vi "Open Hardware.vi"(8 "error in (no error)":errorcluster, 11 "Inst.Krohn-Hite-7008 in":refnum<class "Inst.Krohn-Hite-7008.lvclass">) -> (0 "error out":errorcluster, 3 "Inst.Krohn-Hite-7008 out":refnum<class "Inst.Krohn-Hite-7008.lvclass">)   [LabVIEW 2019, in "Inst.Krohn-Hite-7008.lvclass"]
uses:
  Inst.Krohn-Hite-7008.lvclass
  C:/Program Files (x86)/National Instruments/LabVIEW 2019/user.lib/LevyLab/Instrument Framework/SMOs/Instrument/Instrument.lvclass
  Inst.Krohn-Hite-7008.lvclass/Inst.Krohn-Hite-7008.ctl
  <userlib>/LevyLab/Instrument Framework/SMOs/Instrument/Instrument.lvclass/Instrument.ctl
  <userlib>/LevyLab/Instrument Framework/Instrument Types/VSource/Instrument.VSource.lvclass
  <userlib>/LevyLab/Instrument Framework/SMOs/Instrument/Instrument.lvclass
  <userlib>/LevyLab/D2XX-LV/D2XX-lv.lvlib
  KH7008/KH7008.lvlib
  C:/Program Files (x86)/National Instruments/LabVIEW 2019/user.lib/LevyLab/Instrument Framework/Instrument Types/VSource/Instrument.VSource.lvclass
  C:/Program Files (x86)/National Instruments/LabVIEW 2019/vi.lib/JKI/JKI SMO/SMO/SMO.lvclass
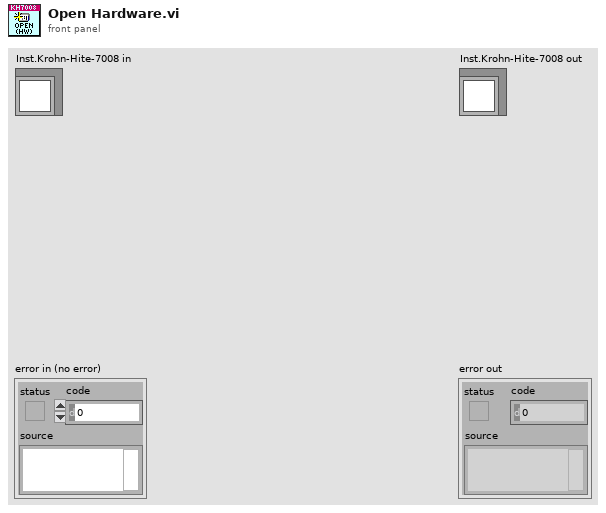
[diagram p1: front panel]
types:
  T1 = typedef "D2XX-lv.lvlib/Device Info.ctl" = cluster{"Serial Number":string, "COM port":string, "Description":string}
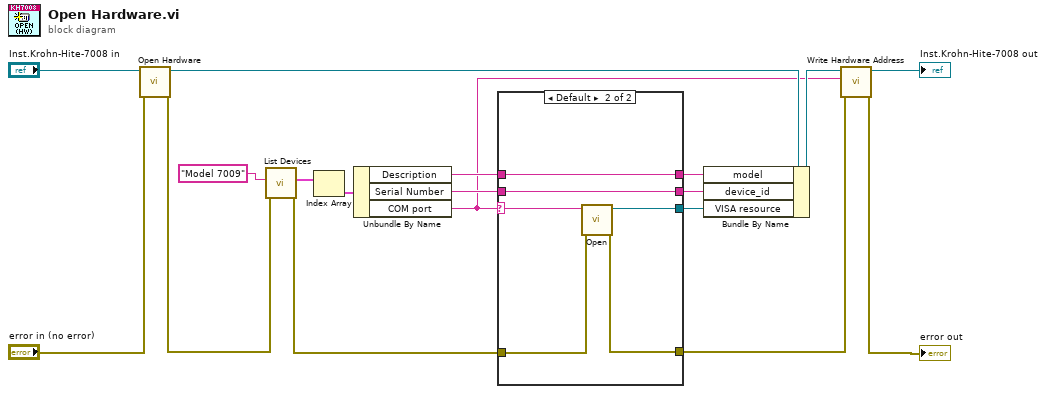
[diagram p0: block diagram]
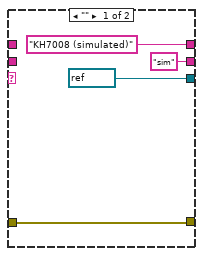
[diagram p2: hidden frame]
diagram:
  n1 = call-parent "Open Hardware.vi"("error in (no error)"="error in (no error)", "Instrument in"="Inst.Krohn-Hite-7008 in") -> ("error out"=w13:errorcluster, "Instrument out"=w16:refnum<class "Inst.Krohn-Hite-7008.lvclass">)  [unwired: 8 in]
  n2 = call <userlib>:"List Devices.vi"("error in (no error)"=w13, "Filter (Device Description)"="Model 7009") -> ("error out"=w11:errorcluster, "Devices"=w7:T1[])  [unwired: 8 in]
  n3 = Index Array(array=w7) -> (element=w6:T1)  [unwired: 1 in]
  n4 = Unbundle By Name(w6) -> ("Description"=w3:string, "Serial Number"=w5:string, "COM port"=w1:string)
  n5 = case shown="Default" w1 {
    selector: w1 -> [_ w26]
    tunnel: w11 -> [w21 w24]
    tunnel: [w21 w23] -> w9
    tunnel: [refnum<visa-resource-name> "sim" ("VISA resource name out") w25] -> w8
    tunnel: w5 -> [_ w28]
    tunnel: ["sim" ("Serial Number") w28] -> w4
    tunnel: w3 -> [_ w27]
    tunnel: ["KH7008 (simulated)" ("Description") w27] -> w2
    frame "" {
    }
    frame Default {
      n6 = call "Open.vi"("error in (no error)"=w24, "VISA resource name"=w26) -> ("error out"=w23:errorcluster, "VISA resource"=w25:refnum<visa-resource-name>)  [unwired: 8 in]
    }
  }
  n7 = Bundle By Name(cluster=w16, "model"=w2, "device_id"=w4, "VISA resource"=w8) -> (w10:refnum<class "Inst.Krohn-Hite-7008.lvclass">)
  n8 = call <userlib>:"Write Hardware Address.vi"("error in (no error)"=w9, "Address"=w1, "Instrument in"=w10) -> ("error out"=→"error out":errorcluster, "Instrument out"=→"Inst.Krohn-Hite-7008 out":refnum<class "Inst.Krohn-Hite-7008.lvclass">)  [unwired: 7 in]
